vi "readHPSettings.vi"(8 "error in (no error)":errorcluster, 11 "Boot in":refnum<class "Boot.lvclass">) -> (0 "error out":errorcluster, 2 "HPSettings":T1, 3 "Boot out":refnum<class "Boot.lvclass">)   [LabVIEW 2016, in "Boot.lvclass"]
uses:
  Boot.lvclass
  DataTypes/Settings/Set/HPSettings.ctl
  Boot.lvclass/Boot.ctl
  Settings/Settings/Setting.lvclass
  DataTypes/Settings/M1M3SupportSettings.lvlib
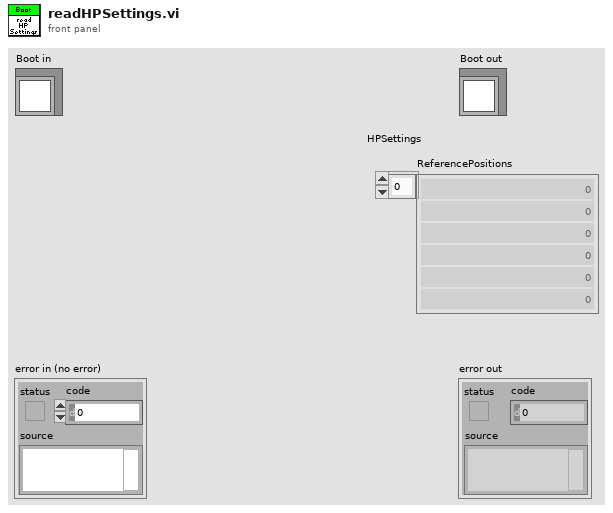
[diagram p1: front panel]
types:
  T1 = typedef "M1M3SupportSettings.lvlib/HPSettings.ctl" = cluster{"ReferencePositions":i32[]}
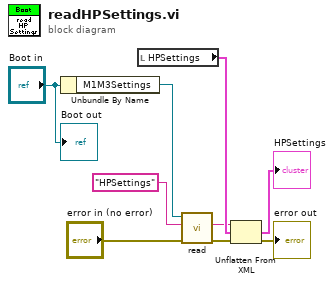
[diagram p0: block diagram]
diagram:
  n1 = Unbundle By Name("Boot in") -> ("M1M3Settings"=w8:refnum<class "Setting.lvclass">)
  n2 = local read "HPSettings"() -> (w7:T1)
  n3 = call-dynamic "read.vi"("error in (no error)"="error in (no error)", "Name"="HPSettings", "BaseSetting in"=w8) -> ("error out"=w1:errorcluster, "XML"=w6:string)  [unwired: 5 in, 2 out]
  n4 = Unflatten From XML(xml string=w6, type=w7, error in (no error)=w1) -> (value=→"HPSettings":T1, error out=→"error out":errorcluster)
  "Boot out" <- "Boot in"
